vi "Create.vi"() -> (8 "Noise":refnum<class "Noise.lvclass">)   [LabVIEW 2020, in "Noise.lvclass"]
uses:
  Noise.lvclass
  Noise.lvclass/Noise.ctl
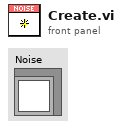
[diagram p1: front panel]
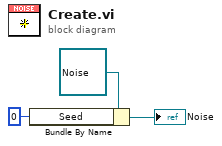
[diagram p0: block diagram]
diagram:
  n1 = Bundle By Name(cluster=refnum<class "Noise.lvclass"> refnum ("Noise"), "Seed"=0 ("Serialized.Seed")) -> (→"Noise":refnum<class "Noise.lvclass">)
